vi "overlay cube numbers.vi"(1 "Circles":cluster{"x":dbl, "y":dbl, "r":dbl}[](array[cluster]), 4 "y 2":dbl[](array[numeric]), 5 "y":dbl[](array[numeric]), 6 "x 2":dbl[](array[numeric]), 7 "Circles 3":cluster{"x":dbl, "y":dbl, "r":dbl}[](array[cluster]), 8 "x":dbl[](array[numeric]), 9 "Image 2":T1(plugin-control)) -> (0 "Circles 4":cluster{"x":dbl, "y":dbl, "r":dbl}[](array[cluster]), 2 "Circles 2":cluster{"x":dbl, "y":dbl, "r":dbl}[](array[cluster]), 3 "Image":T1(plugin-control))   [LabVIEW 2018]
panel:
  out "Y 2":sgl[](array[numeric])
  out "X 2":sgl[](array[numeric])
  out "X":sgl[](array[numeric])
  out "Y":sgl[](array[numeric])
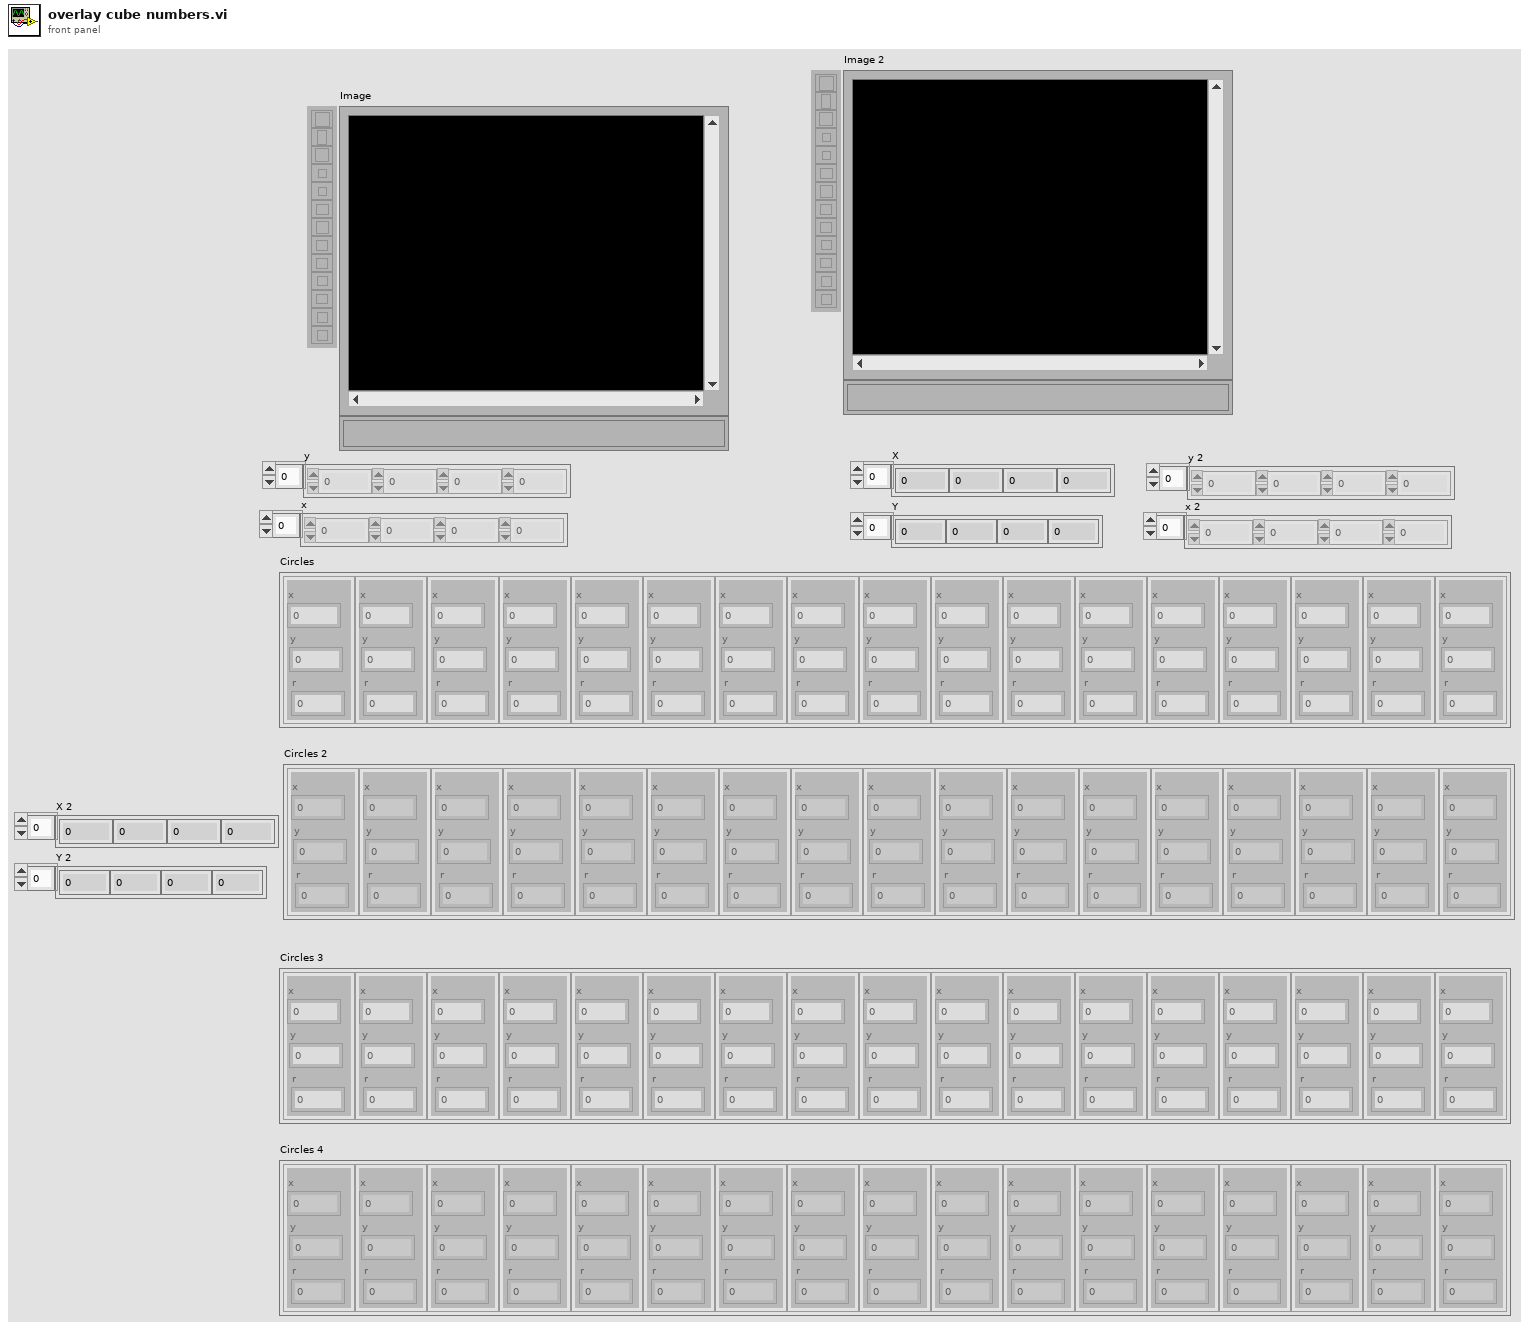
[diagram p1: front panel]
types:
  T1 = typedef "IMAQ Image.ctl" = refnum<image>
  T2 = cluster{"Desired Font (Application)":enum16{"User-specified Font", "Application Font", "System Font", "Dialog Font"}, "[User-specified Font]":cluster{"Font Name":string, "Size":i16, "Strikeout?":bool, "Italic?":bool, "Underline?":bool, "Outline?":bool, "Shadow?":bool, "Bold?":bool, "Rotation Angle":dbl}, "Horizontal Alignment":i16, "Vertical Alignment":i16}
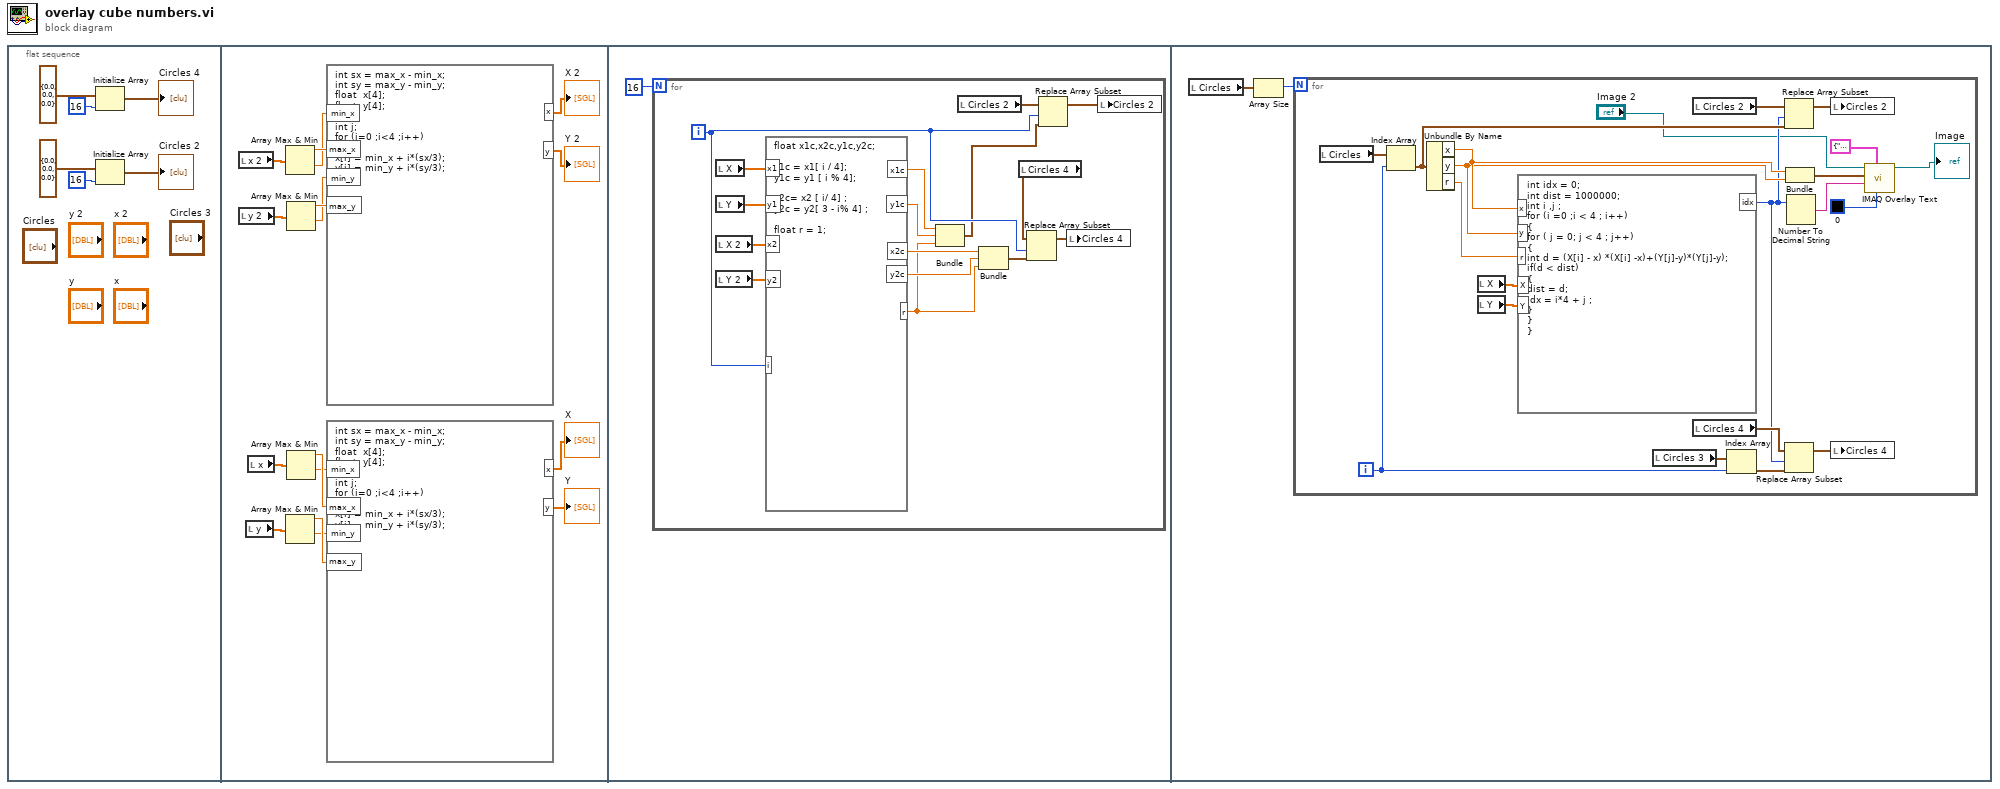
[diagram p0: block diagram]
diagram:
  n1 = flat-sequence {
    frame #0 {
      n2 = Initialize Array(cluster{"x":dbl, "y":dbl, "r":dbl} {"x"=0.0, "y"=0.0, "r"=0.0} ("circle"), 16 ("dimension size")) -> (→"Circles 4":cluster{"x":dbl, "y":dbl, "r":dbl}[])
      n3 = Initialize Array(cluster{"x":dbl, "y":dbl, "r":dbl} {"x"=0.0, "y"=0.0, "r"=0.0} ("circle"), 16 ("dimension size")) -> (→"Circles 2":cluster{"x":dbl, "y":dbl, "r":dbl}[])
    }
    frame #1 {
      n4 = local read "x 2"() -> (w8:dbl[])
      n5 = local read "y 2"() -> (w7:dbl[])
      n6 = local read "y"() -> (w20:dbl[])
      n7 = local read "x"() -> (w19:dbl[])
      n8 = Array Max & Min(array=w8) -> (max value=w12:dbl, min value=w11:dbl)  [unwired: 2 out]
      n9 = Array Max & Min(array=w20) -> (max value=w16:dbl, min value=w15:dbl)  [unwired: 2 out]
      n10 = Array Max & Min(array=w7) -> (max value=w10:dbl, min value=w9:dbl)  [unwired: 2 out]
      n11 = Array Max & Min(array=w19) -> (max value=w18:dbl, min value=w17:dbl)  [unwired: 2 out]
      n12 = formula code="int sx = max_x - min_x;\nint sy = max_y - min_y;\nfloat  x[4];\nfloat  y[4];\nint i;\nint j;\nfor (i=0 ;i<4 ;i++)\n{\nx[i] = min_x + i*(sx/3);\ny[i] = min_y + i*(sy/3);\n}"("min_x"=w11, "max_x"=w12, "min_y"=w9, "max_y"=w10) -> ("x"=→"X 2":dbl[], "y"=→"Y 2":dbl[])
      n13 = formula code="int sx = max_x - min_x;\nint sy = max_y - min_y;\nfloat  x[4];\nfloat  y[4];\nint i;\nint j;\nfor (i=0 ;i<4 ;i++)\n{\nx[i] = min_x + i*(sx/3);\ny[i] = min_y + i*(sy/3);\n}"("min_x"=w17, "max_x"=w18, "min_y"=w15, "max_y"=w16) -> ("x"=→"X":dbl[], "y"=→"Y":dbl[])
    }
    frame #2 {
      n14 = for {
        N: 16 -> [_]
        i -> [w31]
        n15 = local read "X"() -> (w39:sgl[])
        n16 = local read "Y"() -> (w38:sgl[])
        n17 = local read "X 2"() -> (w37:sgl[])
        n18 = local read "Y 2"() -> (w36:sgl[])
        n19 = formula code="float x1c,x2c,y1c,y2c;\n\nx1c = x1[ i / 4];\ny1c = y1 [ i % 4];\n\nx2c= x2 [ i/ 4] ;\ny2c = y2[ 3 - i% 4] ;\n\nfloat r = 1;"("i"=w31, "x1"=w39, "y1"=w38, "x2"=w37, "y2"=w36) -> ("x1c"=w30:dbl, "y1c"=w29:dbl, "x2c"=w28:dbl, "y2c"=w27:dbl, "r"=w25:dbl)
        n20 = Bundle(w30, w29, w25) -> (w24:cluster{dbl, dbl, dbl})  [unwired: 1 in]
        n21 = local read "Circles 2"() -> (w34:cluster{"x":dbl, "y":dbl, "r":dbl}[])
        n22 = Bundle(w28, w27, w25) -> (w26:cluster{dbl, dbl, dbl})  [unwired: 1 in]
        n23 = local read "Circles 4"() -> (w32:cluster{"x":dbl, "y":dbl, "r":dbl}[])
        n24 = Replace Array Subset(array=w32, new element=w26, index=w31) -> (w33:cluster{"x":dbl, "y":dbl, "r":dbl}[])
        n25 = Replace Array Subset(array=w34, new element=w24, index=w31) -> (w35:cluster{"x":dbl, "y":dbl, "r":dbl}[])
        n26 = local write "Circles 4"(w33) -> ()
        n27 = local write "Circles 2"(w35) -> ()
      }
    }
    frame #3 {
      n28 = local read "Circles"() -> (w40:cluster{"x":dbl, "y":dbl, "r":dbl}[])
      n29 = Array Size(array=w40) -> (size(s)=w41:i32)
      n30 = for {
        N: w41 -> [_]
        i -> [w48]
        n31 = local read "Circles"() -> (w62:cluster{"x":dbl, "y":dbl, "r":dbl}[])
        n32 = Index Array(array=w62, index=w48) -> (element=w56:cluster{"x":dbl, "y":dbl, "r":dbl})
        n33 = Unbundle By Name(w56) -> ("x"=w54:dbl, "y"=w53:dbl, "r"=w59:dbl)
        n34 = local read "X"() -> (w61:sgl[])
        n35 = local read "Y"() -> (w60:sgl[])
        n36 = formula code="int idx = 0;\nint dist = 1000000;\nint i ,j ;\nfor (i =0 ;i < 4 ; i++)\n{\nfor ( j = 0; j < 4 ; j++)\n{\nint d = (X[i] - x) *(X[i] -x)+(Y[j]-y)*(Y[j]-y);\nif(d < dist) \n{\ndist = d;\nidx = i*4 + j ;\n}\n}\n}"("x"=w54, "y"=w53, "r"=w59, "X"=w61, "Y"=w60) -> ("idx"=w45:i32)
        n37 = local read "Circles 3"() -> (w49:cluster{"x":dbl, "y":dbl, "r":dbl}[])
        n38 = local read "Circles 2"() -> (w57:cluster{"x":dbl, "y":dbl, "r":dbl}[])
        n39 = local read "Circles 4"() -> (w47:cluster{"x":dbl, "y":dbl, "r":dbl}[])
        n40 = Index Array(array=w49, index=w48) -> (element=w44:cluster{"x":dbl, "y":dbl, "r":dbl})
        n41 = Replace Array Subset(array=w57, new element=w56, index=w45) -> (w58:cluster{"x":dbl, "y":dbl, "r":dbl}[])
        n42 = Replace Array Subset(array=w47, new element=w44, index=w45) -> (w46:cluster{"x":dbl, "y":dbl, "r":dbl}[])
        n43 = Bundle("x"=w54, "y"=w53) -> (w55:cluster{"x":dbl, "y":dbl})  [unwired: 1 in]
        n44 = Number To Decimal String(number=w45) -> (decimal integer string=w52:string)  [unwired: 1 in]
        n45 = local write "Circles 2"(w58) -> ()
        n46 = local write "Circles 4"(w46) -> ()
        n47 = call "IMAQ Overlay Text"("Text Color (black)"=u32 0, "Font, Size & Style"=T2 {"Desired Font (Application)"=enum."User-specified Font", "[User-specified Font]"={"Font Name"="", "Size"=25, "Strikeout?"=FALSE, "Italic?"=FALSE, "Underline?"=TRUE, "Outline?"=FALSE, "Shadow?"=TRUE, "Bold?"=TRUE, "Rotation Angle"=0.0}, "Horizontal Alignment"=1, "Vertical Alignment"=2}, "String"=w52, "Origin"=w55, "Image"="Image 2") -> ("Image Out"=→"Image":T1)  [unwired: 5 in, 1 out]
      }
    }
  }
